vi "Calibration.vi"(3 "Analogue In":refnum<k21>, 5 "Digital In":refnum<k21>) -> (0 "Analogue In Out":refnum<k21>, 1 "Digital Out":refnum<k21>)   [LabVIEW 2016]
uses:
  controls/CalibrationEnum.ctl
  controls/ColourCalibration.ctl
  controls/SettingsEnum.ctl
  controls/PinOut.ctl
  <vilib>/DAQmx/write.llb/DAQmx Write (Digital 1D Bool NChan 1Samp 1Line).vi
  <vilib>/DAQmx/write.llb/DAQmx Write (Analog 1D DBL NChan 1Samp).vi
  <vilib>/DAQmx/miscellaneous.llb/DAQmx Fill In Error Info.vi
  <vilib>/DAQmx/create/channels.llb/DAQmx Create Channel (AO-Voltage-Basic).vi
  <resource>/objmgr/daqmx.rc
panel:
  in  "PushtoController":bool
  in  "Calibration Coordinates":T1 {"Focus Offset /um" min=0.0 max=10.0 step=0.05 scale=-100.0..20.0 scale format="%.2f"; "Colour"."Filter" items=["Empty"=1, ""=2, ""=3, "561"=4, ""=5, "488"=6]}
  in  "Calibration Map":T2
  in  "Piezo Focus /V":dbl(slide)=5.0 scale=0.0..10.0
  out "State":T3=enum."YMirrorVolt"
  in  "stop":bool
  in  "Z Voltage /V":dbl(slide)=-3.815028901734104 scale=-2.0..1.0
  in  "Y Voltage /V":dbl(slide)=2.485549132947977 scale=-5.0..4.0
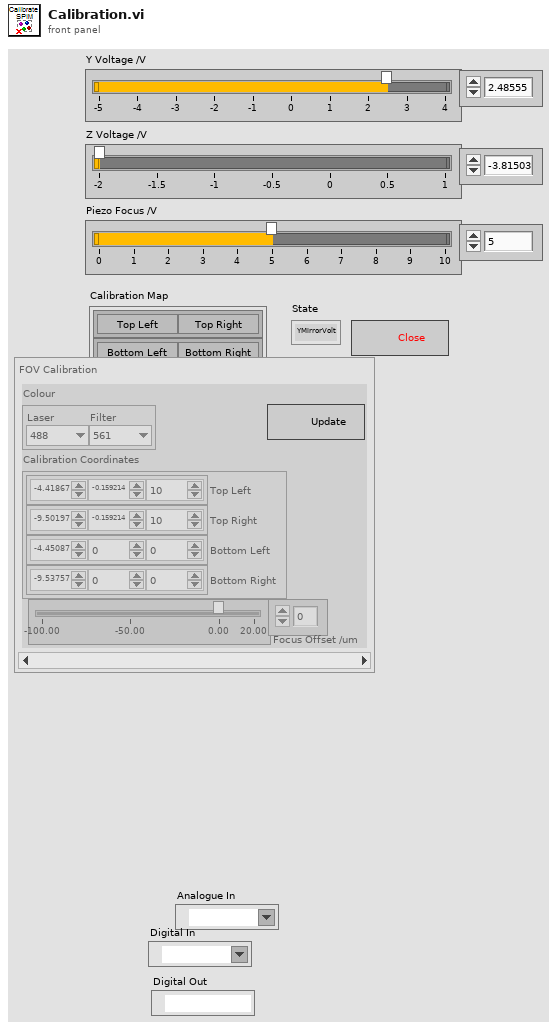
[diagram p1: front panel]
types:
  T1 = typedef "ColourCalibration.ctl" = cluster{"Colour":cluster{"Laser":enum16{"Brightfield", "445", "488", "561", "647"}, "Filter":u16}, "Calibration Coordinates":cluster{"Top Left":dbl[], "Top Right":dbl[], "Bottom Left":dbl[], "Bottom Right":dbl[]}, "Focus Offset /um":dbl}[]
  T2 = cluster{"Cluster 2":cluster{"Top Left":bool, "Top Right":bool}, "Cluster":cluster{"Bottom Left":bool, "Bottom Right":bool}}
  T3 = typedef "CalibrationEnum.ctl" = enum16{"idle", "PiezoVolt", "ColorSwitch", "YMirrorVolt", "ZMirrorVolt", "STOP"}
  T4 = typedef "SettingsEnum.ctl" = enum16{"Idle", "Init", "Calibration Update", "stop"}
  T5 = cluster{"Analogue":refnum<k21>, "Digital":refnum<k21>}
  T6 = cluster{"Colour":cluster{"Laser":enum16{"Brightfield", "445", "488", "561", "647"}, "Filter":u16}, "Calibration Coordinates":cluster{"Top Left":dbl[], "Top Right":dbl[], "Bottom Left":dbl[], "Bottom Right":dbl[]}, "Focus Offset /um":dbl}
  T7 = cluster{"Top Left":dbl[], "Top Right":dbl[], "Bottom Left":dbl[], "Bottom Right":dbl[]}
  T8 = typedef "PinOut.ctl" = string
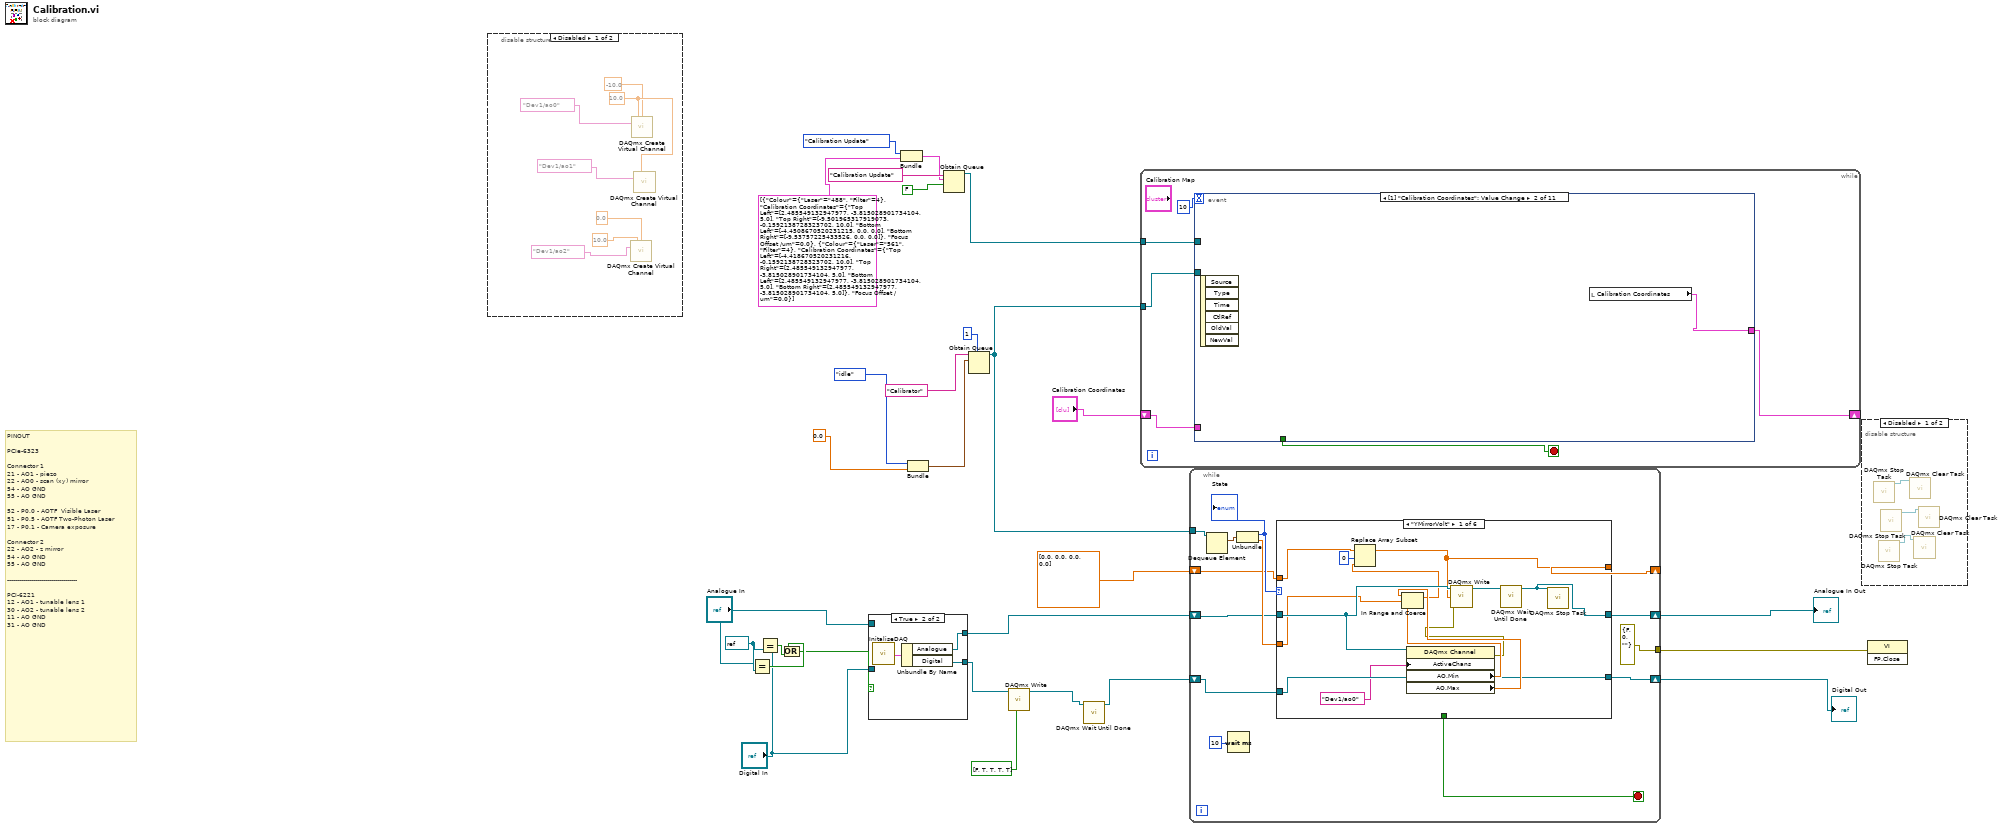
[diagram p0: block diagram]
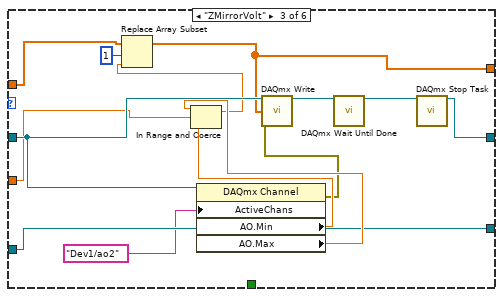
[diagram p6: hidden frame]
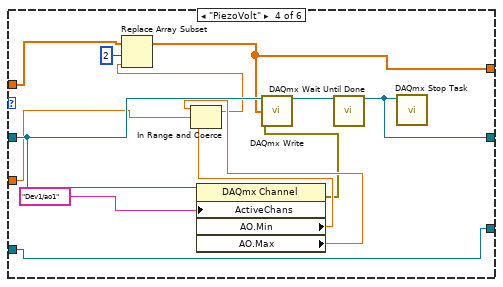
[diagram p7: hidden frame]
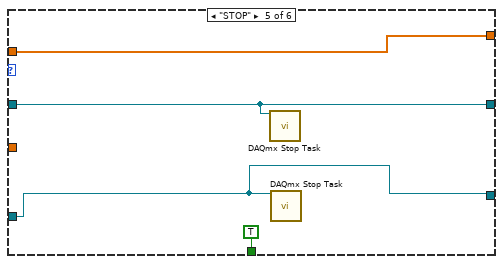
[diagram p8: hidden frame]
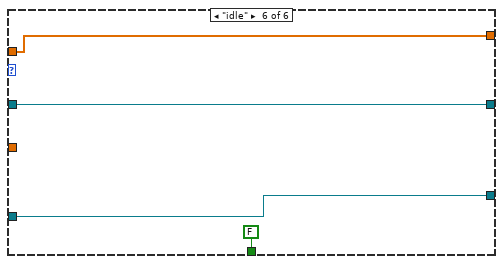
[diagram p9: hidden frame]
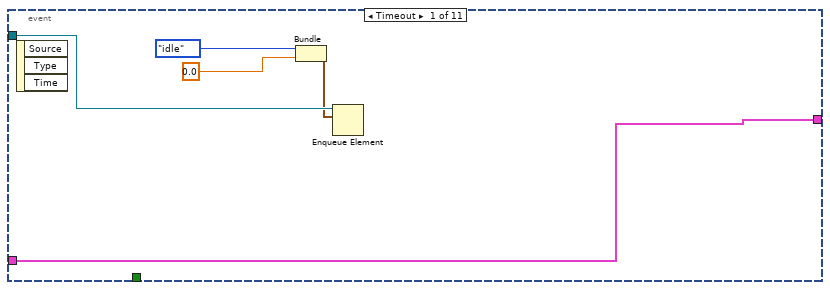
[diagram p10: hidden frame]
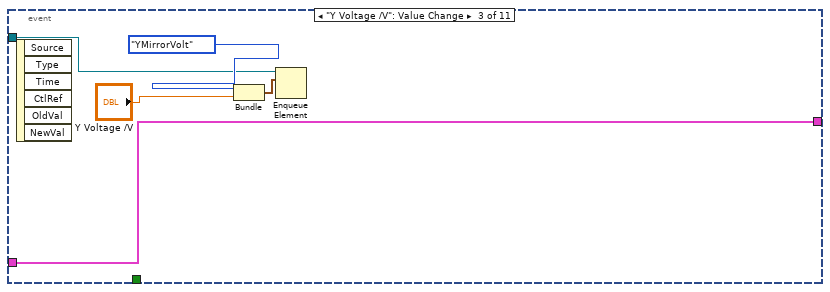
[diagram p11: hidden frame]
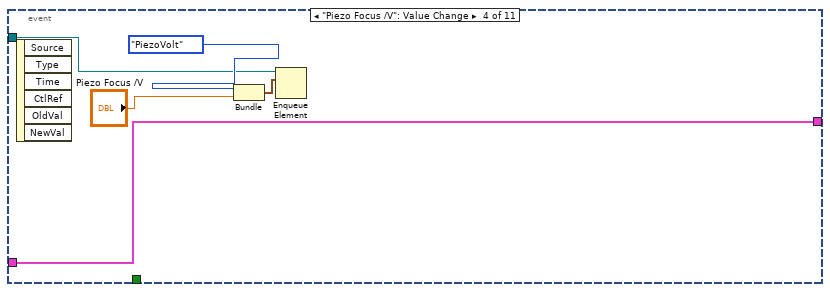
[diagram p12: hidden frame]
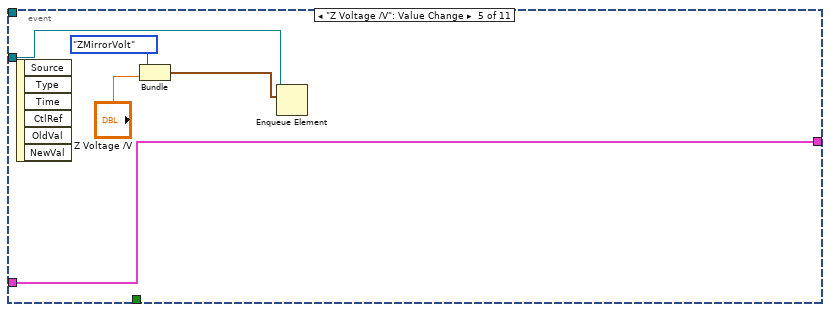
[diagram p13: hidden frame]
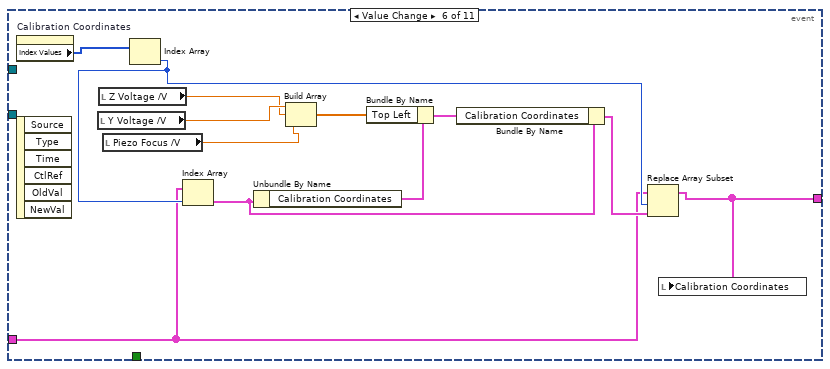
[diagram p14: hidden frame]
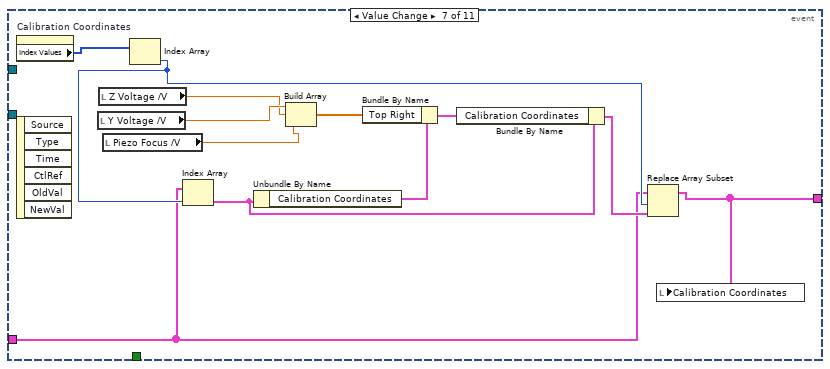
[diagram p15: hidden frame]
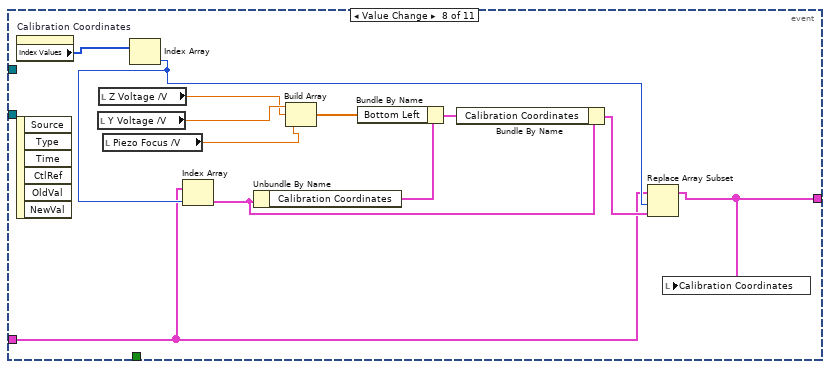
[diagram p16: hidden frame]
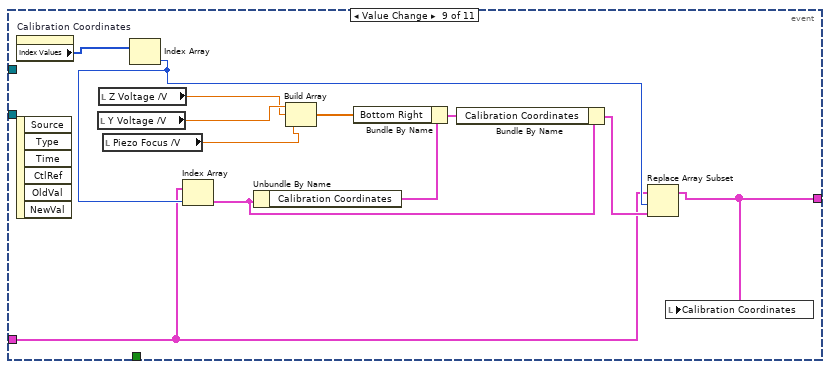
[diagram p17: hidden frame]
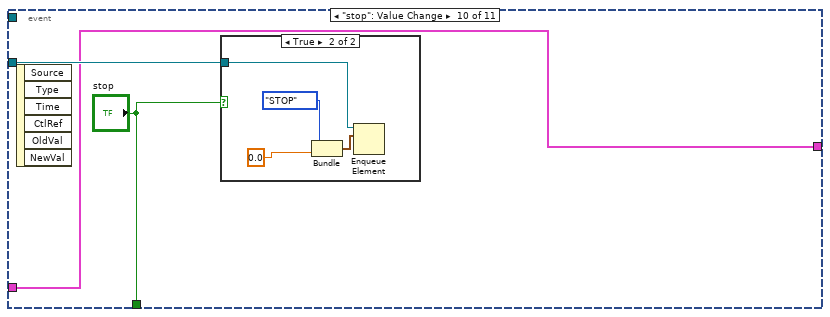
[diagram p18: hidden frame]
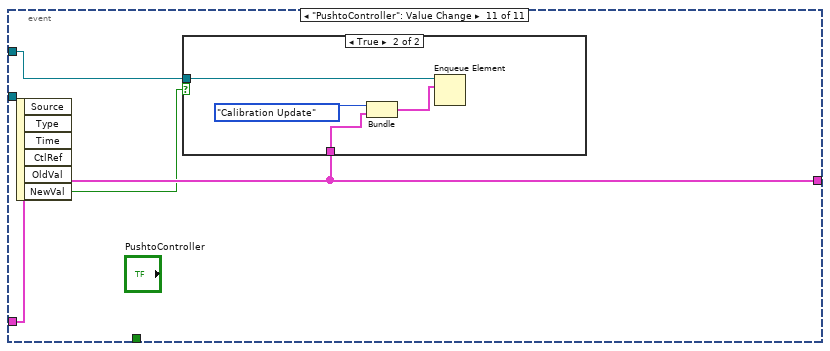
[diagram p20: hidden frame]
diagram:
  w20 = refnum<k21> refnum ("Mirror Y")
  # "PINOUT\n\nPCIe-6323\n\nConnector 1\n21 - AO1 - piezo\n22 - AO0 - scan (xy) mirror\n54 - AO GND\n55 - AO GND\n\n52 - P0.0 - AOTF  Visible Laser\n51 - P0.5 - AOTF Two-Photon Laser\n17 - P0.1 - Camera exposure\n\nConnector 2\n22 - AO2 - z mirror\n54 - AO GND\n55 - AO GND\n\n-----------------------------------\n\nPCI-6221\n12 - AO1 - tunable lens 1\n30 - AO2 - tunable lens 2\n11 - AO GND\n31 - AO GND"
  n1 = disable-structure shown="Disabled" {
    frame Disabled {
      w35 = 10.0 ("maximum value")
      n2 = call-poly <vilib>:"DAQmx Create Virtual Channel.vi"("maximum value"=10.0 ("minimum value"), "minimum value"=0.0 ("maximum value"), "physical channels"=tag "Dev1/ao2") -> ()  [unwired: 11 in, 2 out]
      n3 = call-poly <vilib>:"DAQmx Create Virtual Channel.vi"("maximum value"=w35, "minimum value"=-10.0, "physical channels"=tag "Dev1/ao0") -> ()  [unwired: 11 in, 2 out]
      n4 = call-poly <vilib>:"DAQmx Create Virtual Channel.vi"("maximum value"=w35, "physical channels"=tag "Dev1/ao1") -> ()  [unwired: 12 in, 2 out]
    }
    frame Enabled {
    }
  }
  n5 = Equal?(x="Analogue In", y=w20) -> (x = y?=w18:bool)
  n6 = Equal?(x="Digital In", y=w20) -> (x = y?=w19:bool)
  n7 = Or(x=w18, y=w19) -> (x .or. y?=w17:bool)
  n8 = case shown="True" w17 {
    tunnel: [w37 w38] -> w15
    tunnel: [w36 w39] -> w16
    tunnel: "Digital In" -> [w37 _]
    tunnel: "Analogue In" -> [w36 _]
    frame False {
    }
    frame True {
      n9 = call "InitaliseDAQ.vi"() -> ("Channels"=w40:T5)
      n10 = Unbundle By Name(w40) -> ("Analogue"=w39:refnum<k21>, "Digital"=w38:refnum<k21>)
    }
  }
  n11 = Bundle("Enum"=SettingsEnum."Calibration Update", "Calibration Coordinates"=T1 [{"Colour"={"Laser"=enum."488", "Filter"=4}, "Calibration Coordinates"={"Top Left"=[2.485549132947977, -3.815028901734104, 5.0], "Top Right"=[-9.501965317919073, -0.1592138728323702, 10.0], "Bottom Left"=[-4.4508670520231215, 0.0, 0.0], "Bottom Right"=[-9.53757225433526, 0.0, 0.0]}, "Focus Offset /um"=0.0}, {"Colour"={"Laser"=enum."561", "Filter"=4}, "Calibration Coordinates"={"Top Left"=[-4.418670520231216, -0.1592138728323702, 10.0], "Top Right"=[2.485549132947977, -3.815028901734104, 5.0], "Bottom Left"=[2.485549132947977, -3.815028901734104, 5.0], "Bottom Right"=[2.485549132947977, -3.815028901734104, 5.0]}, "Focus Offset /um"=0.0}]) -> (w1:cluster{"Enum":T4, "Calibration Coordinates":T1})  [unwired: 1 in]
  n12 = Bundle(CalibrationEnum."idle", 0.0) -> (w23:cluster{T3, dbl})  [unwired: 1 in]
  n13 = Obtain Queue(name (unnamed)="Calibration Update", element data type=w1, create if not found? (T)=FALSE) -> (queue out=w7:refnum<queue>)  [unwired: 2 in, 2 out]
  n14 = Obtain Queue(max queue size (-1, unlimited)=1, name (unnamed)="Calibrator", element data type=w23) -> (queue out=w28:refnum<queue>)  [unwired: 2 in, 2 out]
  n15 = call-poly <vilib>:"DAQmx Write.vi"("task/channels in"=w15, "data"=bool[] [FALSE, TRUE, TRUE, TRUE, TRUE]) -> ("task out"=w9:refnum<k21>)  [unwired: 11 in, 2 out]
  n16 = call <vilib>:"DAQmx Wait Until Done.vi"("task/channels in"=w9) -> ("task out"=w8:refnum<k21>)  [unwired: 13 in, 1 out]
  n17 = while {
    tunnel: w28 -> [w45]
    shift-right: [w41] -> _
    shift-left: "Calibration Coordinates" -> [w43]
    tunnel: w7 -> [w42]
    stop <- w44 stop-if-true
    n18 = event shown="[1] \"Calibration Coordinates\": Value Change" {
      selector: _ -> [_ _ _ _ _ _ _ _ _ _ _]
      dyn-events: _ -> [_ _ _ _ _ _ _ _ _ _ _]
      timeout: 10 -> [_ _ _ _ _ _ _ _ _ _ _]
      tunnel: w45 -> [w49 _ w54 w60 w64 _ _ _ _ w118 _]
      tunnel: [_ _ _ _ _ _ _ _ _ "stop" _] -> w44
      tunnel: w43 -> [w47 _ w53 w58 w63 w69 w81 w93 w105 w116 w124]
      tunnel: [w47 w52 w53 w58 w63 w68 w80 w92 w104 w116 w124] -> w41
      tunnel: w42 -> [_ _ _ _ _ _ _ _ _ _ w125]
      event Timeout {
        n19 = event-data() -> ()  [unwired: 1 in, 3 out]
        n20 = Bundle(CalibrationEnum."idle", "minimum value"=0.0) -> (w48:cluster{T3, "minimum value":dbl})  [unwired: 1 in]
        n21 = Enqueue Element(queue=w49, element=w48) -> ()  [unwired: 2 in, 3 out]
      }
      event Value Change {
        n22 = event-data() -> ()  [unwired: 1 in, 6 out]
        n23 = local read "Calibration Coordinates"() -> (w52:T1)
      }
      event "Y Voltage /V": Value Change {
        n24 = event-data() -> ()  [unwired: 1 in, 6 out]
        n25 = Bundle(CalibrationEnum."YMirrorVolt", "Y Voltage /V"="Y Voltage /V") -> (w55:cluster{T3, "Y Voltage /V":dbl})  [unwired: 1 in]
        n26 = Enqueue Element(queue=w54, element=w55) -> ()  [unwired: 2 in, 3 out]
      }
      event "Piezo Focus /V": Value Change {
        n27 = event-data() -> ()  [unwired: 1 in, 6 out]
        n28 = Bundle(CalibrationEnum."PiezoVolt", "Piezo Focus /V"="Piezo Focus /V") -> (w61:cluster{T3, "Piezo Focus /V":dbl})  [unwired: 1 in]
        n29 = Enqueue Element(queue=w60, element=w61) -> ()  [unwired: 2 in, 3 out]
      }
      event "Z Voltage /V": Value Change {
        n30 = event-data() -> ()  [unwired: 1 in, 6 out]
        n31 = Bundle(CalibrationEnum."ZMirrorVolt", "Z Voltage /V"="Z Voltage /V") -> (w65:cluster{T3, "Z Voltage /V":dbl})  [unwired: 1 in]
        n32 = Enqueue Element(queue=w64, element=w65) -> ()  [unwired: 2 in, 3 out]
      }
      event "Calibration Map.Cluster 2.Top Left": Value Change {
        n33 = property on="Calibration Coordinates" class="Arr (strict)"() -> ("Index Values"=w76:u32[])  [unwired: 2 in, 2 out]
        n34 = event-data() -> ()  [unwired: 1 in, 6 out]
        n35 = local read "Y Voltage /V"() -> (w79:dbl)
        n36 = local read "Z Voltage /V"() -> (w78:dbl)
        n37 = local read "Piezo Focus /V"() -> (w77:dbl)
        n38 = Index Array(array=w76) -> (element=w74:u32)  [unwired: 1 in]
        n39 = Index Array(array=w69, index=w74) -> (element=w72:T6)
        n40 = Unbundle By Name(w72) -> ("Calibration Coordinates"=w73:T7)
        n41 = Build Array(w79, w78, w77) -> (w75:dbl[])
        n42 = Bundle By Name(cluster=w73, "Top Left"=w75) -> (w71:T7)
        n43 = Bundle By Name(cluster=w72, "Calibration Coordinates"=w71) -> (w70:T6)
        n44 = Replace Array Subset(array=w69, new element=w70, index=w74) -> (w68:T1)
        n45 = local write "Calibration Coordinates"(w68) -> ()
      }
      event "Calibration Map.Cluster 2.Top Right": Value Change {
        n46 = property on="Calibration Coordinates" class="Arr (strict)"() -> ("Index Values"=w88:u32[])  [unwired: 2 in, 2 out]
        n47 = event-data() -> ()  [unwired: 1 in, 6 out]
        n48 = local read "Y Voltage /V"() -> (w91:dbl)
        n49 = local read "Z Voltage /V"() -> (w90:dbl)
        n50 = local read "Piezo Focus /V"() -> (w89:dbl)
        n51 = Index Array(array=w88) -> (element=w86:u32)  [unwired: 1 in]
        n52 = Index Array(array=w81, index=w86) -> (element=w84:T6)
        n53 = Unbundle By Name(w84) -> ("Calibration Coordinates"=w85:T7)
        n54 = Build Array(w91, w90, w89) -> (w87:dbl[])
        n55 = Bundle By Name(cluster=w85, "Top Right"=w87) -> (w83:T7)
        n56 = Bundle By Name(cluster=w84, "Calibration Coordinates"=w83) -> (w82:T6)
        n57 = Replace Array Subset(array=w81, new element=w82, index=w86) -> (w80:T1)
        n58 = local write "Calibration Coordinates"(w80) -> ()
      }
      event "Calibration Map.Cluster.Bottom Left": Value Change {
        n59 = property on="Calibration Coordinates" class="Arr (strict)"() -> ("Index Values"=w100:u32[])  [unwired: 2 in, 2 out]
        n60 = event-data() -> ()  [unwired: 1 in, 6 out]
        n61 = local read "Y Voltage /V"() -> (w103:dbl)
        n62 = local read "Z Voltage /V"() -> (w102:dbl)
        n63 = local read "Piezo Focus /V"() -> (w101:dbl)
        n64 = Index Array(array=w100) -> (element=w98:u32)  [unwired: 1 in]
        n65 = Index Array(array=w93, index=w98) -> (element=w96:T6)
        n66 = Unbundle By Name(w96) -> ("Calibration Coordinates"=w97:T7)
        n67 = Build Array(w103, w102, w101) -> (w99:dbl[])
        n68 = Bundle By Name(cluster=w97, "Bottom Left"=w99) -> (w95:T7)
        n69 = Bundle By Name(cluster=w96, "Calibration Coordinates"=w95) -> (w94:T6)
        n70 = Replace Array Subset(array=w93, new element=w94, index=w98) -> (w92:T1)
        n71 = local write "Calibration Coordinates"(w92) -> ()
      }
      event "Calibration Map.Cluster.Bottom Right": Value Change {
        n72 = property on="Calibration Coordinates" class="Arr (strict)"() -> ("Index Values"=w112:u32[])  [unwired: 2 in, 2 out]
        n73 = event-data() -> ()  [unwired: 1 in, 6 out]
        n74 = local read "Y Voltage /V"() -> (w115:dbl)
        n75 = local read "Z Voltage /V"() -> (w114:dbl)
        n76 = local read "Piezo Focus /V"() -> (w113:dbl)
        n77 = Index Array(array=w112) -> (element=w110:u32)  [unwired: 1 in]
        n78 = Index Array(array=w105, index=w110) -> (element=w108:T6)
        n79 = Unbundle By Name(w108) -> ("Calibration Coordinates"=w109:T7)
        n80 = Build Array(w115, w114, w113) -> (w111:dbl[])
        n81 = Bundle By Name(cluster=w109, "Bottom Right"=w111) -> (w107:T7)
        n82 = Bundle By Name(cluster=w108, "Calibration Coordinates"=w107) -> (w106:T6)
        n83 = Replace Array Subset(array=w105, new element=w106, index=w110) -> (w104:T1)
        n84 = local write "Calibration Coordinates"(w104) -> ()
      }
      event "stop": Value Change {
        n85 = event-data() -> ()  [unwired: 1 in, 6 out]
        n86 = case shown="True" "stop" {
          tunnel: w118 -> [_ w122]
          frame False {
          }
          frame True {
            n87 = Bundle(CalibrationEnum."STOP", "minimum value"=0.0) -> (w119:cluster{T3, "minimum value":dbl})  [unwired: 1 in]
            n88 = Enqueue Element(queue=w122, element=w119) -> ()  [unwired: 2 in, 3 out]
          }
        }
      }
      event "PushtoController": Value Change {
        n89 = event-data() -> ("NewVal"=w123:bool)  [unwired: 1 in, 5 out]
        n90 = case shown="True" w123 {
          tunnel: w125 -> [_ w129]
          tunnel: w124 -> [_ w127]
          frame False {
          }
          frame True {
            n91 = Bundle("Enum"=SettingsEnum."Calibration Update", "Calibration Coordinates"=w127) -> (w126:cluster{"Enum":T4, "Calibration Coordinates":T1})  [unwired: 1 in]
            n92 = Enqueue Element(queue=w129, element=w126) -> ()  [unwired: 2 in, 3 out]
          }
        }
      }
    }
  }
  n93 = while {
    tunnel: w28 -> [w142]
    shift-right: [w138] -> w12
    shift-left: w16 -> [w139]
    shift-right: [w134] -> _
    shift-left: dbl[] [0.0, 0.0, 0.0, 0.0] -> [w135]
    shift-right: [w132] -> w11
    shift-left: w8 -> [w133]
    tunnel: [errorcluster {"status"=FALSE, "code"=0, "source"=""} ("error out")] -> w10
    stop <- w137 stop-if-true
    n94 = Dequeue Element(queue=w142) -> (element=w141:cluster{T3, dbl})  [unwired: 2 in, 3 out]
    n95 = Wait (ms)(milliseconds to wait=u32 10) -> ()  [unwired: 1 out]
    n96 = Unbundle(w141) -> (w136:T3, w140:dbl)
    "State" <- w136
    n97 = case shown="\"YMirrorVolt\"" w136 {
      tunnel: w140 -> [w151 _ w168 w181 _ _]
      tunnel: w139 -> [w154 w158 w171 w184 w188 w192]
      tunnel: [w144 w158 w160 w174 w188 w192] -> w138
      tunnel: [_ _ _ _ TRUE ("stop") FALSE ("stop")] -> w137
      tunnel: w135 -> [w149 w157 w166 w179 w189 w191]
      tunnel: [w147 w157 w164 w177 w189 w191] -> w134
      tunnel: w133 -> [w145 w156 w162 w175 w186 w190]
      tunnel: [w145 w156 w162 w175 w186 w190] -> w132
      frame "YMirrorVolt" {
        n98 = property class="DAQmx Channel"(reference=w154, "ActiveChans"=T8 "Dev1/ao0" ("Combo Box")) -> (error out=w146:errorcluster, "AO.Min"=w153:dbl, "AO.Max"=w152:dbl)  [unwired: 1 in, 1 out]
        n99 = In Range and Coerce(upper limit=w152, x=w151, lower limit=w153) -> (coerced(x)=w148:dbl)  [unwired: 1 out]
        n100 = Replace Array Subset(array=w149, new element=w148, index=0) -> (w147:dbl[])
        n101 = call-poly <vilib>:"DAQmx Write.vi"("task/channels in"=w154, "data"=w147, "error in"=w146) -> ("task out"=w155:refnum<k21>)  [unwired: 10 in, 2 out]
        n102 = call <vilib>:"DAQmx Wait Until Done.vi"("task/channels in"=w155) -> ("task out"=w144:refnum<k21>)  [unwired: 13 in, 1 out]
        n103 = call <vilib>:"DAQmx Stop Task.vi"("task/channels in"=w144) -> ()  [unwired: 13 in, 2 out]
      }
      frame "ColorSwitch" {
      }
      frame "ZMirrorVolt" {
        n104 = property class="DAQmx Channel"(reference=w171, "ActiveChans"=T8 "Dev1/ao2" ("Combo Box")) -> (error out=w163:errorcluster, "AO.Min"=w170:dbl, "AO.Max"=w169:dbl)  [unwired: 1 in, 1 out]
        n105 = In Range and Coerce(upper limit=w169, x=w168, lower limit=w170) -> (coerced(x)=w165:dbl)  [unwired: 1 out]
        n106 = Replace Array Subset(array=w166, new element=w165, index=1) -> (w164:dbl[])
        n107 = call-poly <vilib>:"DAQmx Write.vi"("task/channels in"=w171, "data"=w164, "error in"=w163) -> ("task out"=w172:refnum<k21>)  [unwired: 10 in, 2 out]
        n108 = call <vilib>:"DAQmx Wait Until Done.vi"("task/channels in"=w172) -> ("task out"=w161:refnum<k21>)  [unwired: 13 in, 1 out]
        n109 = call <vilib>:"DAQmx Stop Task.vi"("task/channels in"=w161) -> ("task out"=w160:refnum<k21>)  [unwired: 13 in, 1 out]
      }
      frame "PiezoVolt" {
        n110 = property class="DAQmx Channel"(reference=w184, "ActiveChans"=T8 "Dev1/ao1" ("Combo Box")) -> (error out=w176:errorcluster, "AO.Min"=w183:dbl, "AO.Max"=w182:dbl)  [unwired: 1 in, 1 out]
        n111 = In Range and Coerce(upper limit=w182, x=w181, lower limit=w183) -> (coerced(x)=w178:dbl)  [unwired: 1 out]
        n112 = Replace Array Subset(array=w179, new element=w178, index=2) -> (w177:dbl[])
        n113 = call-poly <vilib>:"DAQmx Write.vi"("task/channels in"=w184, "data"=w177, "error in"=w176) -> ("task out"=w185:refnum<k21>)  [unwired: 10 in, 2 out]
        n114 = call <vilib>:"DAQmx Wait Until Done.vi"("task/channels in"=w185) -> ("task out"=w174:refnum<k21>)  [unwired: 13 in, 1 out]
        n115 = call <vilib>:"DAQmx Stop Task.vi"("task/channels in"=w174) -> ()  [unwired: 13 in, 2 out]
      }
      frame "STOP" {
        n116 = call <vilib>:"DAQmx Stop Task.vi"("task/channels in"=w188) -> ()  [unwired: 13 in, 2 out]
        n117 = call <vilib>:"DAQmx Stop Task.vi"("task/channels in"=w186) -> ()  [unwired: 13 in, 2 out]
      }
      frame "idle" {
      }
    }
  }
  "Analogue In Out" <- w12
  "Digital Out" <- w11
  n118 = disable-structure shown="Disabled" {
    frame Disabled {
      n119 = call <vilib>:"DAQmx Stop Task.vi"() -> ("task out"=w196:refnum<k21>)  [unwired: 14 in, 1 out]
      n120 = call <vilib>:"DAQmx Stop Task.vi"() -> ("task out"=w194:refnum<k21>)  [unwired: 14 in, 1 out]
      n121 = call <vilib>:"DAQmx Stop Task.vi"() -> ("task out"=w195:refnum<k21>)  [unwired: 14 in, 1 out]
      n122 = call <vilib>:"DAQmx Clear Task.vi"("task in"=w196) -> ()  [unwired: 14 in, 1 out]
      n123 = call <vilib>:"DAQmx Clear Task.vi"("task in"=w194) -> ()  [unwired: 14 in, 1 out]
      n124 = call <vilib>:"DAQmx Clear Task.vi"("task in"=w195) -> ()  [unwired: 14 in, 1 out]
    }
    frame Enabled {
    }
  }
  n125 = invoke class="VI" method="FP.Close"(error in=w10) -> ()  [unwired: 2 in, 3 out]
